vi "Extract Profile Array.vi"(8 "error in (no error)":errorcluster caption="エラー入力 (エラーなし)", 9 "Profile Cnt":u32, 10 "Profile Data":u32[](array[numeric]), 11 "Profile Info":T1) -> (0 "error out":errorcluster caption="エラー出力", 1 "Luminance Profile Array":u16[][](array[numeric]), 2 "16位forImage":i16[][](array[numeric]), 3 "Header Array":u32[][](array[numeric]))   [LabVIEW 2015, in "KEYENCE LJ-X8000A.lvlib"]
doc: "Only height data of profiles without a header and footer will be extracted to output in two-dimensional array from profile data acquired with VI such as <B>Read Profiles</B> VI.\n\n<B>Note</B>:\nEmpty array will be output for corresponding output data if there is no profile data to extract."
uses:
  KEYENCE LJ-X8000A.lvlib
  Clusters/Profile Info.ctl
panel:
  out "Height Profile Array":dbl[][](array[numeric])
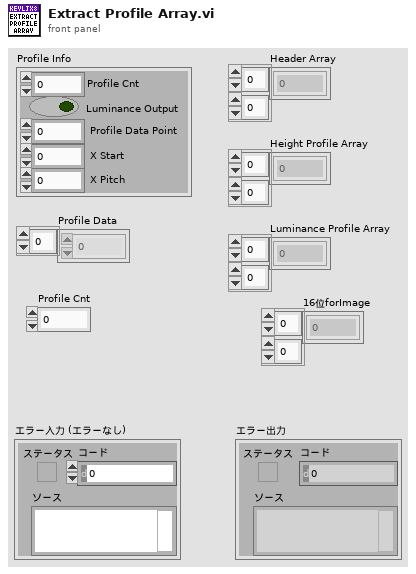
[diagram p1: front panel]
types:
  T1 = typedef "KEYENCE LJ-X8000A.lvlib/Profile Info.ctl" = cluster{"Profile Cnt":u8, "Luminance Output":bool, " Profile Data Point":u16, " X Start":i32, " X Pitch":i32}
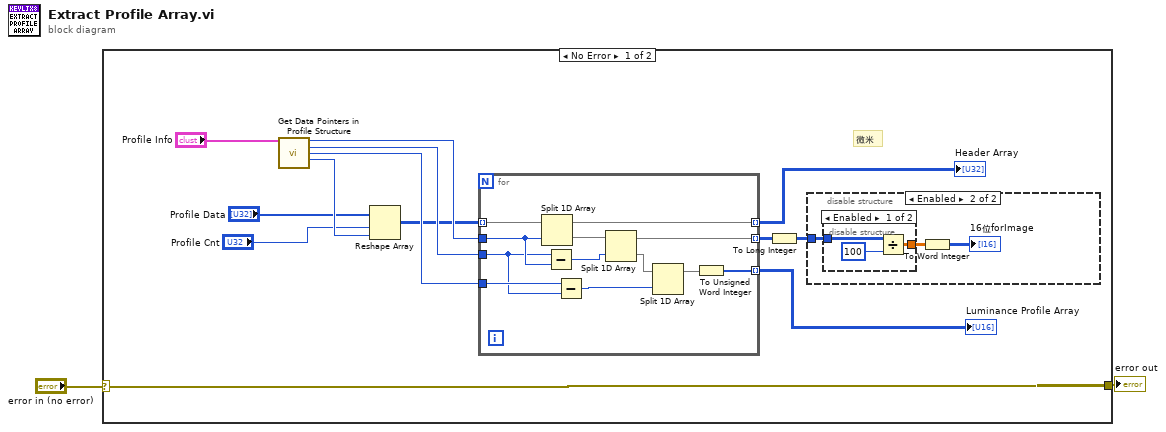
[diagram p0: block diagram]
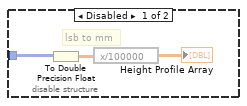
[diagram p2: hidden frame]
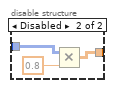
[diagram p3: hidden frame]
diagram:
  n1 = case shown="No Error" "error in (no error)" {
    selector: "error in (no error)" -> [w5 w40]
    tunnel: [w5 w40] -> w1
    frame No Error {
      # "微米"
      n2 = call "Get Data Pointers in Profile Structure.vi"("Profile Info"="Profile Info") -> ("Height Profile Pointer Index"=w9:u32, "Luminance Profile Pointer Index"=w13:u32, "Footer Pointer Index"=w14:u32, "Data Num of Raw Profile Structure"=w10:u32)  [unwired: 10 in, 1 out]
      n3 = Reshape Array("Profile Data", "Profile Cnt", w10) -> (w8:u32[][])
      n4 = for {
        tunnel: w8 -> [w39] mode=indexing
        tunnel: w9 -> [w35]
        tunnel: w13 -> [w33]
        tunnel: [w37] -> w11 mode=indexing
        tunnel: [w31] -> w15 mode=indexing
        tunnel: [w28] -> w12 mode=indexing
        tunnel: w14 -> [w34]
        n5 = Split 1D Array(array=w39, index=w35) -> (first subarray=w37:u32[], second subarray=w38:u32[])
        n6 = Subtract(x=w33, y=w35) -> (x-y=w36:u32)
        n7 = Subtract(x=w34, y=w33) -> (x-y=w32:u32)
        n8 = Split 1D Array(array=w38, index=w36) -> (first subarray=w31:u32[], second subarray=w30:u32[])
        n9 = Split 1D Array(array=w30, index=w32) -> (first subarray=w29:u32[])  [unwired: 1 out]
        n10 = To Unsigned Word Integer(number=w29) -> (unsigned 16bit integer=w28:u16[])
      }
      "Luminance Profile Array" <- w12
      "Header Array" <- w11
      n11 = To Long Integer(number=w15) -> (32bit integer=w3:i32[][])
      n12 = disable-structure shown="Enabled" {
        disable-tunnel: w3 -> [w18 w21]
        frame Disabled {
          # "lsb to mm"
          n13 = To Double Precision Float(number=w18) -> (double precision float=w16:dbl[][])
          n14 = expression code="x/100000"(w16) -> (→"Height Profile Array":dbl[][])
        }
        frame Enabled {
          n15 = disable-structure shown="Enabled" {
            disable-tunnel: w21 -> [w24 w27]
            disable-tunnel: [w22 w25] -> w20
            frame Enabled {
              n16 = Divide(x=w24, y=100) -> (x/y=w22:dbl[][])
            }
            frame Disabled {
              n17 = Multiply(x=w27, y=0.8) -> (x*y=w25:dbl[][])
            }
          }
          n18 = To Word Integer(number=w20) -> (16bit integer=→"16位forImage":i16[][])
        }
      }
    }
    frame Error {
    }
  }
  "error out" <- w1
